vi "testfifort.vi"() -> ()   [LabVIEW 2010]
uses:
  <vilib>/rvi/interface/nirviOpenFPGA/nirviOpenFPGA.xnode
  C:/Users/HAGAR-IV/Desktop/Zeugs/Johnny/pertrasgc fpga/testfifoeinzeln.vi
  <vilib>/userDefined/High Color/nirio_resource_hc.ctl
  <vilib>/rvi/interface/nirviMethod/nirviMethod.xnode
  <vilib>/rvi/interface/nirviReadWriteControl/nirviReadWriteControl.xnode
  <vilib>/rvi/errors/niLvFpgaWhatHappensToTopLevelVI.ctl
  <vilib>/rvi/interface/common/niFpgaNodeNameForErrorReporting.ctl
  <vilib>/rvi/errors/niLvFpgaAdjustHostInterfaceError.vi
  <vilib>/rvi/interface/nirviCloseFPGA/nirviCloseFPGA.xnode
  <vilib>/RVI Host/nirviSupport.llb/nirviErrorClusterFromErrorCode.vi
  <vilib>/FPGAPlugInAG/cRIO-9114/niLvFpga_Close_cRIO-9114.vi
panel:
  out "Data":fxp<+/-,26,5>[](array[numeric]) format="%.23g"
  out "x-y":u32
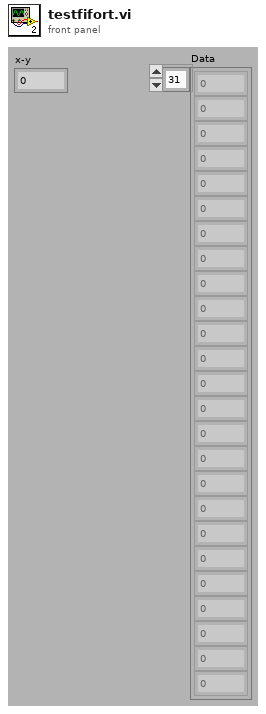
[diagram p1: front panel]
types:
  T1 = typedef "niFpgaNodeNameForErrorReporting.ctl" = enum16{"Open FPGA VI Reference", "Read/Write Control", "Invoke Method: Abort", "Invoke Method: Acknowledge IRQ", "Invoke Method: Download", "Invoke Method: FIFO.Configure", "Invoke Method: FIFO.Read", "Invoke Method: FIFO.Start", "Invoke Method: FIFO.Stop", "Invoke Method: FIFO.Write", "Invoke Method: Reset", "Invoke Method: Run", "Invoke Method: Wait on IRQ", "Close FPGA VI Reference"}
  T2 = typedef "niLvFpgaWhatHappensToTopLevelVI.ctl" = enum16{"top level VI scripted behind XNode", "top level VI inlined behind XNode"}
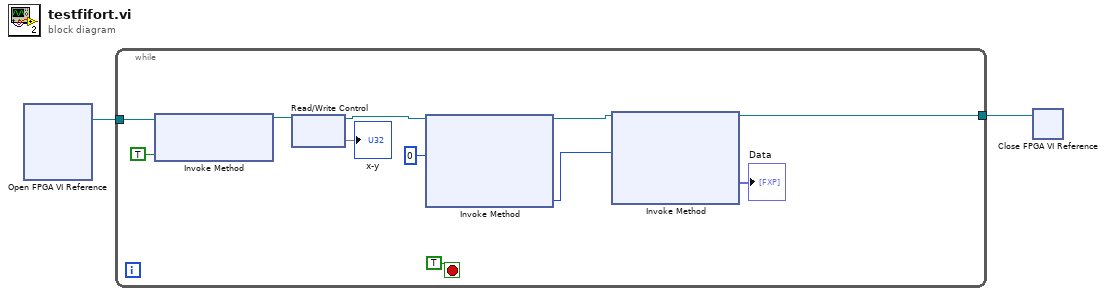
[diagram p0: block diagram]
diagram:
  n1 = xnode "Open FPGA VI Reference"() -> ("FPGA VI Reference Out"=w2:refnum<k20>)  [unwired: 2 in, 1 out]
  n2 = while {
    tunnel: w2 -> [w12]
    tunnel: [w3] -> w1
    stop <- TRUE ("Stopp") stop-if-true
    n3 = xnode "Invoke Method"("FPGA VI Reference In"=w12, "Wait Until Done (F)"=TRUE) -> ("FPGA VI Reference Out"=w10:refnum<k20>)  [unwired: 1 in, 1 out]
    n4 = xnode "Read/Write Control"("FPGA VI Reference In"=w10) -> ("FPGA VI Reference Out"=w8:refnum<k20>, "x-y"=→"x-y")  [unwired: 1 in, 1 out]
    n5 = xnode "Invoke Method"("FPGA VI Reference In"=w8, "Number of Elements"=u32 0) -> ("FPGA VI Reference Out"=w6:refnum<k20>, "Elements Remaining"=w5:u32)  [unwired: 2 in, 2 out]
    n6 = xnode "Invoke Method"("FPGA VI Reference In"=w6, "Number of Elements"=w5) -> ("FPGA VI Reference Out"=w3:refnum<k20>, "Data"=→"Data":fxp<+/-,26,5>[])  [unwired: 2 in, 2 out]
  }
  n7 = xnode "Close FPGA VI Reference"("FPGA VI Reference In"=w1) -> ()  [unwired: 1 in, 1 out]
